vi "FRCts20_Backend_INI_Write_DB_String.vi"(8 "error in (no error)":errorcluster, 9 "Save? (T)":bool=TRUE, 10 "Connection String":string="Driver={MySQL ODBC 5.2w Driver};Server=parkway-test-db.cjlclmebggwl.us-east-1.rds.amazonaws.com", 11 "INI Controller in":refnum<class "FRCts20_Backend_INI Controller.lvclass">) -> (0 "error out":errorcluster, 3 "INI Controller out":refnum<class "FRCts20_Backend_INI Controller.lvclass">)   [LabVIEW 2014, in "FRCts20_Backend_Engine.lvlib" / "FRCts20_Backend_INI Controller.lvclass"]
uses:
  FRCts20_Backend_INI Controller.lvclass
  FRCts20_Backend_INI Controller.lvclass/FRCts20_Backend_INI Controller.ctl
  <vilib>/Utility/config.llb/Write Key (String).vi
  <vilib>/Utility/config.llb/NI_LVConfig.lvlib
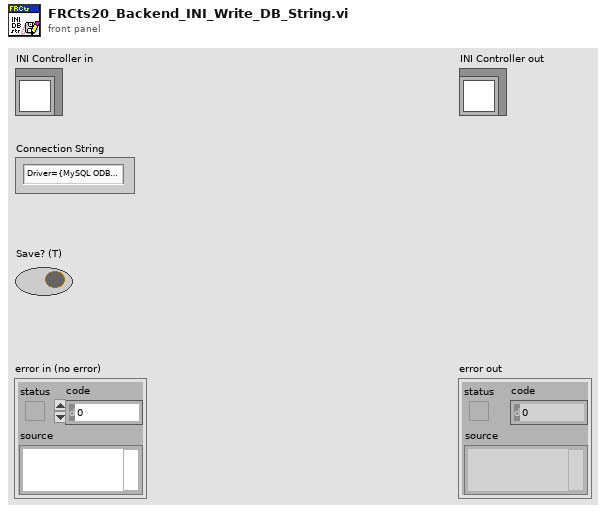
[diagram p1: front panel]
types:
  T1 = typedef "NI_LVConfig.lvlib/Config Data RefNum.ctl" = refnum<k1>
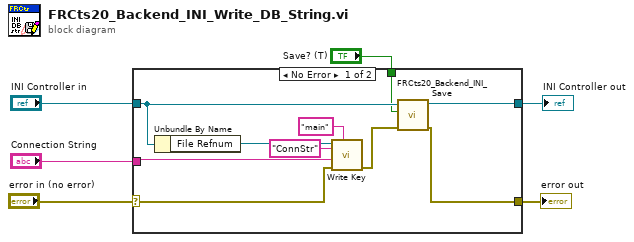
[diagram p0: block diagram]
diagram:
  n1 = case shown="No Error" "error in (no error)" {
    selector: "error in (no error)" -> [w10 w17]
    tunnel: [w16 w17] -> w5
    tunnel: [w15 w18] -> w3
    tunnel: "INI Controller in" -> [w13 w18]
    tunnel: "Connection String" -> [w7 _]
    tunnel: "Save? (T)" -> [w12 _]
    frame No Error {
      n2 = Unbundle By Name(w13) -> ("File Refnum"=w8:T1)
      n3 = call-poly <vilib>:"Write Key.vi"("section"="main", "error in (no error)"=w10, "value"=w7, "key"="ConnStr", "refnum"=w8) -> ("error out"=w11:errorcluster)  [unwired: 4 in, 2 out]
      n4 = call "FRCts20_Backend_INI_Save.vi"("error in (no error)"=w11, "Save? (T)"=w12, "INI Controller in"=w13) -> ("error out"=w16:errorcluster, "INI Controller out"=w15:refnum<class "FRCts20_Backend_INI Controller.lvclass">)  [unwired: 7 in]
    }
    frame Error {
    }
  }
  "error out" <- w5
  "INI Controller out" <- w3
